vi "Torque Testing.vi"(0 "VISA resource name":refnum<visa-resource-name>="COM13", 1 "Baud Rate":u32=115200, 2 "Data Bits":u16=8 min=5 max=8 step=1, 3 "Parity":u16(ring) items=["None", "Odd", "Even", "Mark", "Space"], 4 "Stop Bits":u16(ring)=10 items=["1.0"=10, "1.5"=15, "2.0"=20], 7 "Flow Control":u16(ring) items=["None"=0, "XON/XOFF"=1, "RTS/CTS"=2, "DTR/DSR"=4]) -> ()   [LabVIEW 2016]
doc: "The Basic Serial Read and Write example performs a Serial Port Read, a Serial Port Write, or a combination of these actions. The user selects the actions (read or write) on the front panel. If both are selected, the VI will write the data first, read data, and then close the VISA session that is opened to the port. This VI will wait until the specified number of bytes is received at the port. Only the number of bytes specified will be read.\n\nINSTRUCTIONS:\n1) Select the serial resource and configuration parameters (baud rate, data bits, parity, stop bits, flow control).\n2) Select the operations to be performed. \n3) Connect the serial port to your device. If no device is available, perform a loopback test by doing one of the following. Short pins 2 and 3 on a RS-232 cable or short pin 4 to pin 8 and pin 5 to pin 9 on a RS-485/422 cable. \n4) Run the VI to see the data read. (The \"read string\" will match the \"string to write\" if a loopback test was performed.)\n\nNote: The parameters set for the serial port must match the parameters of the connected instrument or device. In this example, the bytes to read parameter specifies the number of bytes that the serial port reads. If there were more bytes at the port than the number specified in bytes to read, those bytes would not be read. Also, if you specify to read more bytes than the number of bytes actually read, you might receive a timeout error message.\n\nOn the block diagram, the Configure Serial Port VI sets the configuration parameters. The front panel displays the controls used to configure the basic parameters, such as baud rate, data bits, and parity. Constants configure the other parameters the user probably does not need set. After the VISA Configure Serial Port VI opens the VISA session and configures the port, the VI passes the VISA resource name to other VIs that perform operations on that VISA resource. The VISA Write function sends a command to the serial device and the VISA Read function returns data based on the command. The VISA Close function then closes the reference to the serial device. It is important to close the reference; otherwise communication through with that port through protocols other than VISA might not be possible."
uses:
  <vilib>/Utility/file.llb/Write Delimited Spreadsheet (string).vi
  <vilib>/Utility/file.llb/Write Delimited Spreadsheet (DBL).vi
  <vilib>/Instr/_visa.llb/VISA Configure Serial Port (Instr).vi
panel:
  in  "Start":bool
  out "Path":path
  out "Consumer Loop":dbl
  out "Elements in Queue":dbl format="%#_13g"
  out "XY Graph":cluster{"Y":dbl[], "Y":dbl[]}[](graph)
  out "Cons. Speed":u32
  out "Data":dbl[][](array[numeric])
  out "Items in Queue":i32
  in  "Apply":bool
  out "Iterations / Sec.":dbl
  out "Elapsed Time (sec)":dbl
  out "Iterations":i32
  in  "stop":bool
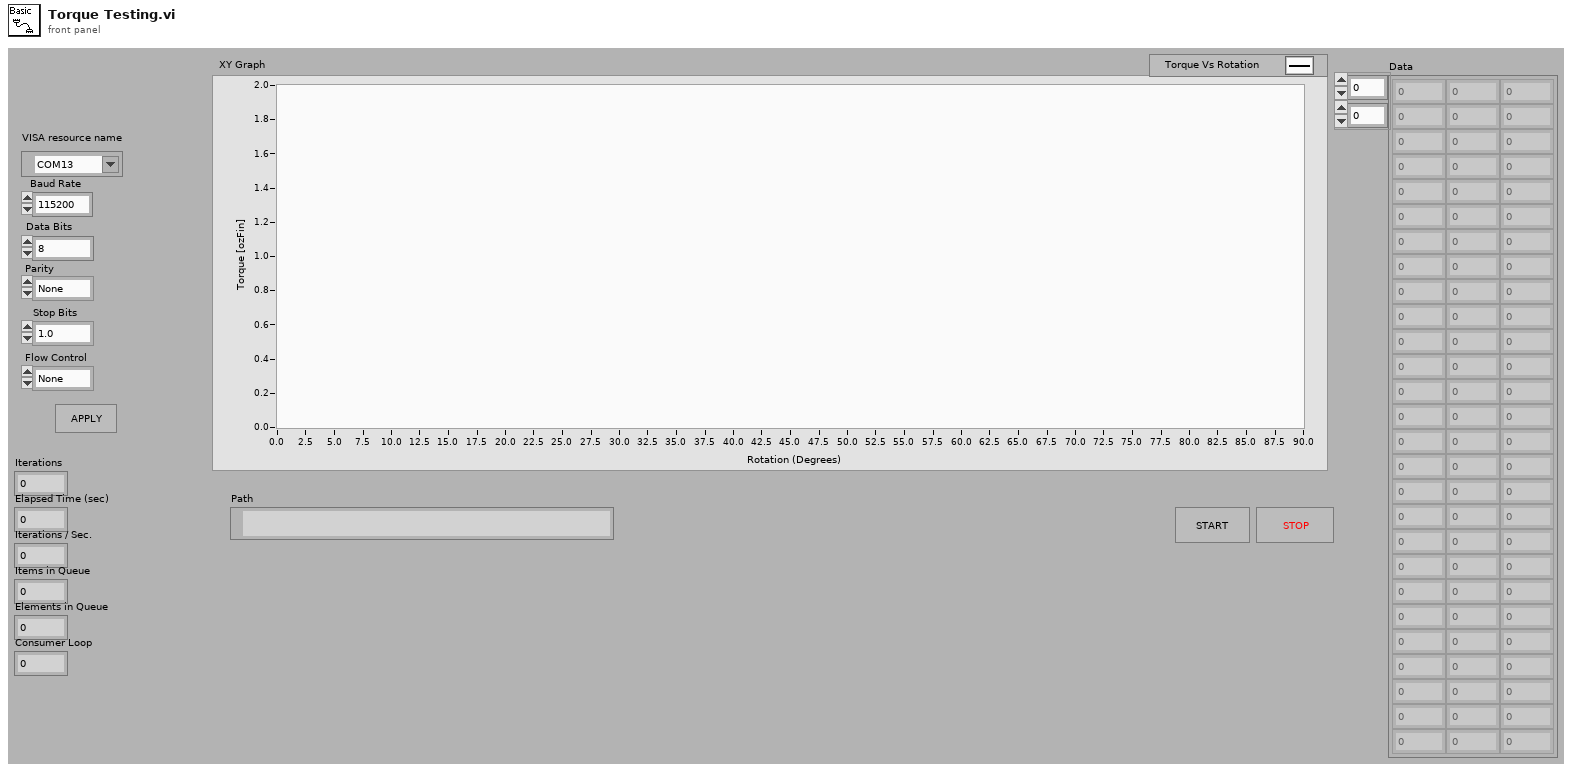
[diagram p1: front panel]
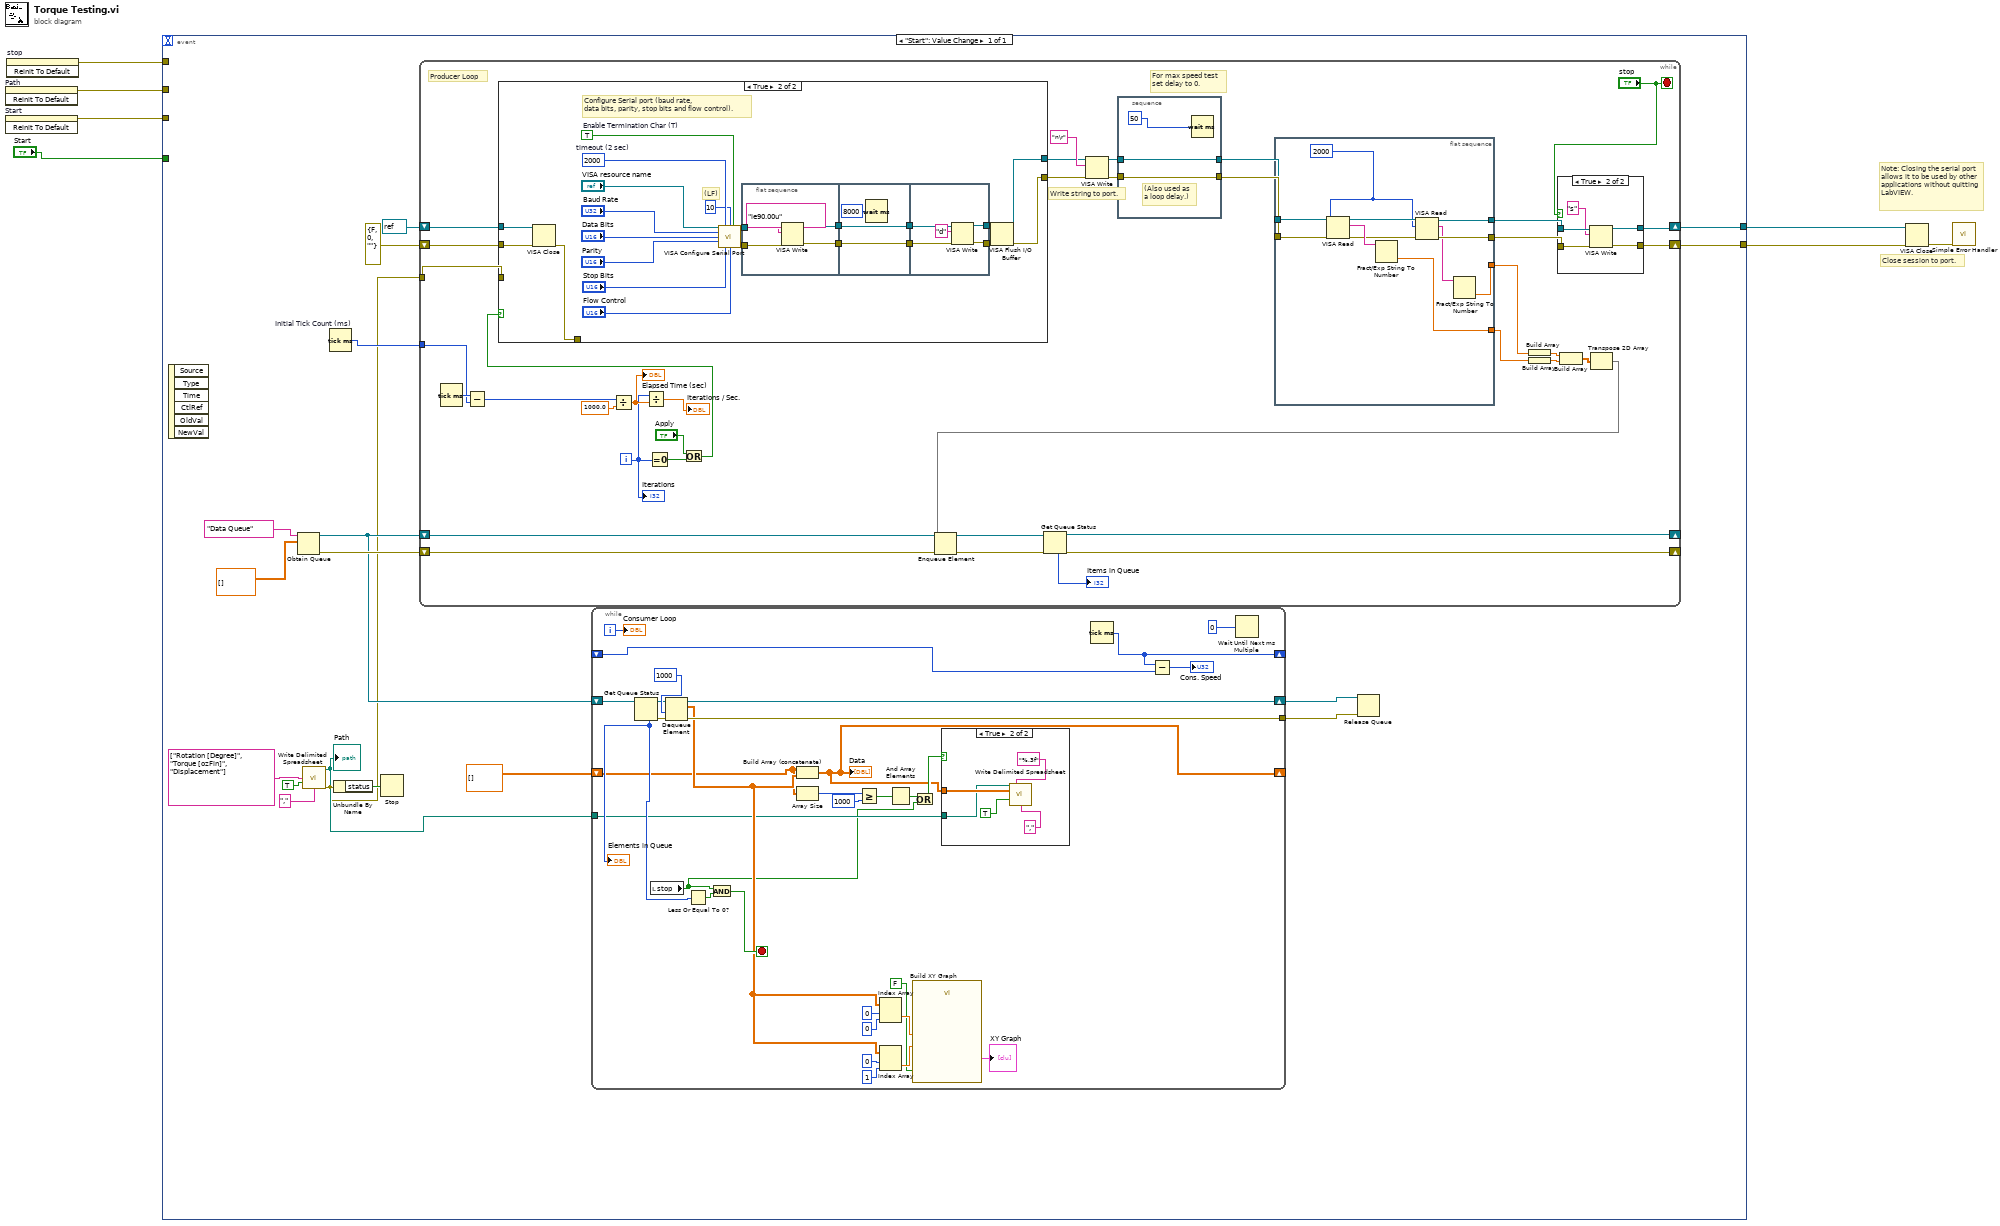
[diagram p0: block diagram]
diagram:
  # "Note: Closing the serial port allows it to be used by other applications without quitting LabVIEW."
  # "Close session to port."
  n1 = invoke on="Path" class="Path" method="Reinit To Default"() -> (error out=w2:errorcluster)  [unwired: 3 in, 2 out]
  n2 = invoke on="Start" class="Bool" method="Reinit To Default"() -> (error out=w1:errorcluster)  [unwired: 3 in, 2 out]
  n3 = invoke on="stop" class="Bool (strict)" method="Reinit To Default"() -> (error out=w3:errorcluster)  [unwired: 3 in, 2 out]
  n4 = event shown="[0] \"Start\": Value Change" {
    selector: _ -> [_]
    dyn-events: _ -> [_]
    timeout: _ -> [_]
    tunnel: [w25] -> w6
    tunnel: [w22] -> w5
    tunnel: "Start" -> [_]
    tunnel: w3 -> [_]
    tunnel: w2 -> [_]
    tunnel: w1 -> [_]
    event "Start": Value Change {
      n5 = event-data() -> ()  [unwired: 1 in, 6 out]
      n6 = Obtain Queue(name (unnamed)="Data Queue", element data type=dbl[][] []) -> (queue out=w18:refnum<queue>, error out=w19:errorcluster)  [unwired: 3 in, 1 out]
      n7 = call-poly <vilib>:"Write Delimited Spreadsheet.vi"("1D data"=string[] ["Rotation [Degree]", "Torque [ozFin]", "Displacement"], "append to file? (new file:F)"=TRUE, "delimiter (\\t)"=",") -> ("new file path (Not A Path if cancelled)"=w13:path, "error out"=w10:errorcluster)  [unwired: 11 in]
      "Path" <- w13
      n8 = Tick Count (ms) "Initial Tick Count (ms)"() -> (millisecond timer value=w24:u32)
      n9 = Unbundle By Name(w10) -> ("status"=w17:bool)
      n10 = Stop(stop? (T)=w17) -> ()
      n11 = while {
        tunnel: w24 -> [w93]
        shift-right: [w71] -> w25
        shift-left: refnum<visa-resource-name> refnum ("VISA resource name out") -> [w89]
        shift-right: [w69] -> w22
        shift-left: errorcluster {"status"=FALSE, "code"=0, "source"=""} ("error out") -> [w88]
        shift-right: [w74] -> _
        shift-left: w18 -> [w80]
        shift-right: [w73] -> _
        shift-left: w19 -> [w79]
        tunnel: w10 -> [w65]
        i -> [w85]
        stop <- "stop" stop-if-true
        # "Producer Loop"
        # "Write string to port."
        # "For max speed test \nset delay to 0."
        n12 = Tick Count (ms) ("Current Tick Count (ms)")() -> (millisecond timer value=w96:u32)
        n13 = Subtract(x=w96, y=w93) -> (x-y=w95:u32)
        n14 = Divide(x=w95, y=1000.0) -> (x/y=w91:dbl)
        "Elapsed Time (sec)" <- w91
        n15 = Divide(x=w85, y=w91) -> (x/y=→"Iterations / Sec.":dbl)
        n16 = Equal To 0?(x=w85) -> (x = 0?=w86:bool)
        n17 = Or(x="Apply", y=w86) -> (x .or. y?=w87:bool)
        n18 = case shown="True" w87 {
          tunnel: [w120 w126] -> w67
          tunnel: [w119 w125] -> w66
          tunnel: w89 -> [w120 w133]
          tunnel: w88 -> [w119 w131]
          tunnel: [_ w132] -> _
          tunnel: w65 -> [_ _]
          frame False {
          }
          frame True {
            w138 = TRUE  # Enable Termination Char (T)
            w139 = u32 2000  # timeout (2 sec)
            # "(LF)"
            # "Configure Serial port (baud rate,\ndata bits, parity, stop bits and flow control)."
            n19 = VISA Close(VISA resource name=w133, error in (no error)=w131) -> (error out=w132:errorcluster)
            n20 = call-poly "VISA Configure Serial Port"("VISA resource name"="VISA resource name", "timeout (10sec)"=w139, "termination char\n(0xA = '\\n' = LF)"=u8 10 ("termination char\n(0xA = '\\n' = LF)"), "Enable Termination\nChar (T)"=w138, "baud rate (9600)"="Baud Rate", "data bits (8)"="Data Bits", "parity (0:none)"="Parity", "stop bits (10: 1 bit)"="Stop Bits", "flow control (0:none)"="Flow Control") -> ("VISA resource name out"=w130:refnum<visa-resource-name>, "error out"=w129:errorcluster)  [unwired: 5 in]
            n21 = flat-sequence {
              tunnel: w130 -> [w147]
              tunnel: w129 -> [w146]
              tunnel: [w145] -> w124
              tunnel: [w144] -> w123
              tunnel: w124 -> [w150]
              tunnel: w123 -> [w149]
              tunnel: [w150] -> w122
              tunnel: [w149] -> w121
              tunnel: [w152] -> w127
              tunnel: [w154] -> w128
              tunnel: w122 -> [w155]
              tunnel: w121 -> [w153]
              frame #0 {
                n22 = VISA Write(VISA resource name=w147, write buffer="ie90.00u", error in (no error)=w146) -> (VISA resource name out=w145:refnum<visa-resource-name>, error out=w144:errorcluster)  [unwired: 1 out]
              }
              frame #1 {
                n23 = Wait (ms)(milliseconds to wait=u32 8000) -> ()  [unwired: 1 out]
              }
              frame #2 {
                n24 = VISA Write(VISA resource name=w155, write buffer="d", error in (no error)=w153) -> (VISA resource name out=w154:refnum<visa-resource-name>, error out=w152:errorcluster)  [unwired: 1 out]
              }
            }
            n25 = VISA Flush I/O Buffer(VISA resource name=w128, error in (no error)=w127) -> (VISA resource name out=w126:refnum<visa-resource-name>, error out=w125:errorcluster)  [unwired: 1 in]
          }
        }
        n26 = VISA Write(VISA resource name=w67, write buffer="n\r" ("String to Write"), error in (no error)=w66) -> (VISA resource name out=w98:refnum<visa-resource-name>, error out=w100:errorcluster)  [unwired: 1 out]
        n27 = stacked-sequence {
          tunnel: w100 -> [w158]
          tunnel: [w158] -> w99
          tunnel: w98 -> [w157]
          tunnel: [w157] -> w97
          frame #0 {
            # "(Also used as\na loop delay.)"
            n28 = Wait (ms)(milliseconds to wait=u32 50 ("t")) -> ()  [unwired: 1 out]
          }
        }
        n29 = flat-sequence {
          tunnel: w99 -> [w118]
          tunnel: w97 -> [w117]
          tunnel: [w116] -> w72
          tunnel: [w115] -> w70
          tunnel: [w109] -> w64
          tunnel: [w108] -> w63
          frame #0 {
            w111 = u32 2000 ("byte count")
            n30 = VISA Read(VISA resource name=w117, byte count=w111, error in (no error)=w118) -> (VISA resource name out=w113:refnum<visa-resource-name>, read buffer=w114:string, error out=w112:errorcluster)  [unwired: 1 out]
            n31 = Fract/Exp String To Number(string=w114) -> (number=w109:dbl)  [unwired: 3 in, 1 out]
            n32 = VISA Read(VISA resource name=w113, byte count=w111, error in (no error)=w112) -> (VISA resource name out=w116:refnum<visa-resource-name>, read buffer=w110:string, error out=w115:errorcluster)  [unwired: 1 out]
            n33 = Fract/Exp String To Number(string=w110) -> (number=w108:dbl)  [unwired: 3 in, 1 out]
          }
        }
        n34 = Build Array(w63) -> (w83:dbl[])
        n35 = Build Array(w64) -> (w82:dbl[])
        n36 = case shown="True" "stop" {
          tunnel: w72 -> [w102 w105]
          tunnel: w70 -> [w101 w107]
          tunnel: [w101 w106] -> w69
          tunnel: [w102 w104] -> w71
          frame False {
          }
          frame True {
            n37 = VISA Write(VISA resource name=w105, write buffer="s", error in (no error)=w107) -> (VISA resource name out=w104:refnum<visa-resource-name>, error out=w106:errorcluster)  [unwired: 1 out]
          }
        }
        n38 = Build Array(w83, w82) -> (w81:dbl[][])
        n39 = Transpose 2D Array(2D array=w81) -> (transposed array=w78:dbl[][])
        n40 = Enqueue Element(queue=w80, element=w78, error in (no error)=w79) -> (queue out=w77:refnum<queue>, error out=w76:errorcluster)  [unwired: 1 in, 1 out]
        n41 = Get Queue Status(queue=w77, error in (no error)=w76) -> (queue out=w74:refnum<queue>, error out=w73:errorcluster, # elements in queue=→"Items in Queue":i32)  [unwired: 1 in, 5 out]
        "Iterations" <- w85
      }
      n42 = while {
        shift-right: [w44] -> w12
        shift-left: w18 -> [w55]
        tunnel: [w45] -> w11
        shift-right: [w34] -> _
        shift-left: _ -> [w33]
        tunnel: w13 -> [w29]
        shift-right: [w27] -> _
        shift-left: dbl[][] [] -> [w26]
        i -> [w57]
        stop <- w52 stop-if-true
        n43 = Get Queue Status(queue=w55) -> (queue out=w43:refnum<queue>, error out=w56:errorcluster, # elements in queue=w51:i32)  [unwired: 2 in, 5 out]
        "Elements in Queue" <- w51
        n44 = local read "stop"() -> (w28:bool)
        n45 = Dequeue Element(queue=w43, timeout in ms (-1)=1000, error in (no error)=w56) -> (queue out=w44:refnum<queue>, element=w30:dbl[][], error out=w45:errorcluster)  [unwired: 1 out]
        n46 = Less Or Equal To 0?(x=w51) -> (x <= 0?=w53:bool)
        n47 = And(x=w28, y=w53) -> (x .and. y?=w52:bool)
        n48 = Build Array (concatenate) ("Data Buffer")(w26, w30) -> (w27:dbl[][])
        "Data" <- w27
        n49 = Array Size(array=w26) -> (size(s)=w49:i32[])
        n50 = Greater Or Equal?(x=w49, y=1000) -> (x >= y?=w31:bool[])
        n51 = Index Array(array=w30, index (row)=0, index (col)=0) -> (element=w39:dbl)
        n52 = Index Array(array=w30, index (row)=0, index (col)=1) -> (element=w36:dbl)
        n53 = And Array Elements(Boolean array=w31) -> (logical AND=w47:bool)
        n54 = call "Build XY Graph"("Reset"=FALSE, "Y Input"=w36, "X Input"=w39) -> ("XY Graph"=→"XY Graph":cluster{"X":dbl[], "Y":dbl[]}[])  [unwired: 7 in, 1 out]
        n55 = Or(x=w47, y=w28) -> (x .or. y?=w46:bool)
        n56 = case shown="True" w46 {
          tunnel: w27 -> [_ w59]
          tunnel: w29 -> [_ w58]
          frame False {
          }
          frame True {
            n57 = call-poly <vilib>:"Write Delimited Spreadsheet.vi"("file path (dialog if empty)"=w58, "format (%.3f)"="%.3f", "2D data"=w59, "append to file? (new file:F)"=TRUE, "delimiter (\\t)"=",") -> ()  [unwired: 9 in, 2 out]
          }
        }
        n58 = Tick Count (ms)() -> (millisecond timer value=w34:u32)
        n59 = Subtract(x=w34, y=w33) -> (x-y=→"Cons. Speed":u32)
        n60 = Wait Until Next ms Multiple(millisecond multiple=0) -> ()  [unwired: 1 out]
        "Consumer Loop" <- w57
      }
      n61 = Release Queue(queue=w12, error in (no error)=w11) -> ()  [unwired: 1 in, 3 out]
    }
  }
  n62 = VISA Close(VISA resource name=w6, error in (no error)=w5) -> (error out=w7:errorcluster)
  n63 = call <vilib>:"Simple Error Handler.vi"("error in (no error)"=w7) -> ()  [unwired: 4 in, 5 out]
